vi "SRV_Determine Incoming Data Type.vi"(0 "Data":string, 11 "error in (no error)":errorcluster) -> (4 "Data dup":string, 10 "Response Data Type":T1=enum."No Data", 15 "error out":errorcluster)   [LabVIEW 2009]
doc: "Searches for identifying characters at the beginning of Data to determine the type of response the data is from.\n\n\nAuthor: Mike Schultz - Logic PD"
uses:
  SRV_Response Data Type.ctl
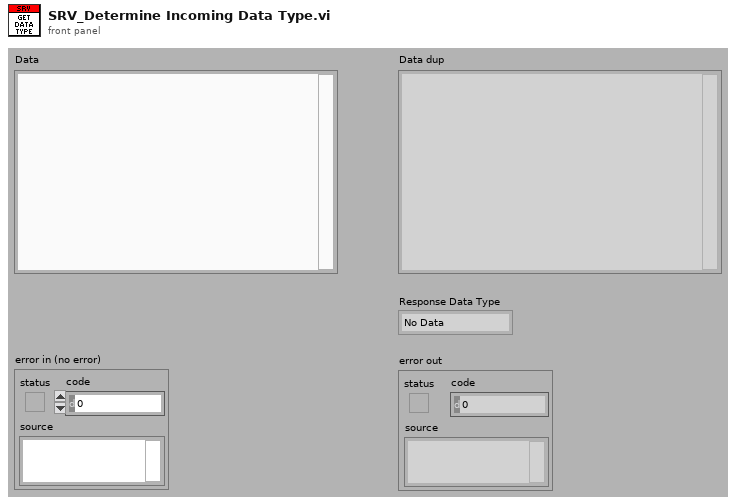
[diagram p1: front panel]
types:
  T1 = typedef "SRV_Response Data Type.ctl" = enum16{"Undefined Data", "##IMJ", "#B", "Leaving PicoC", "##vp", "##zZ", "##N$B", "##N$b", "##i$l", "##i$L", "##i$N", "##&NP,", "##&R,", "No Data"}
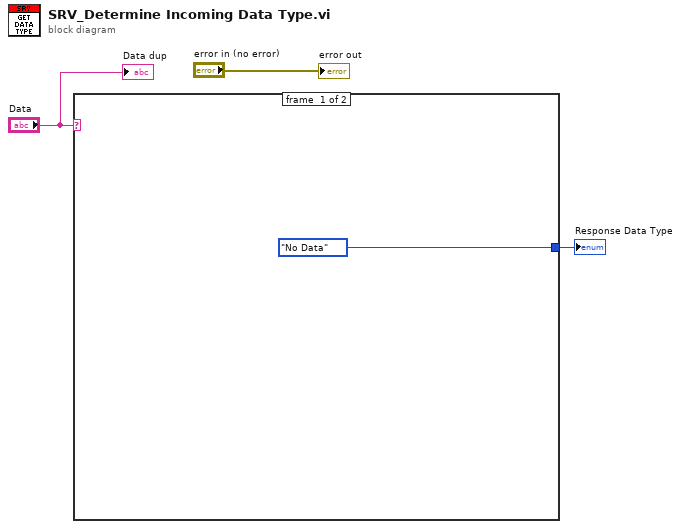
[diagram p0: block diagram]
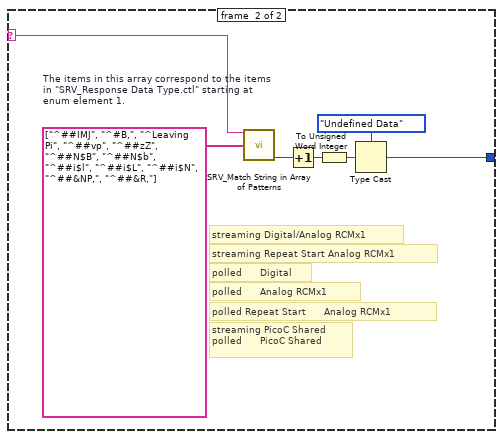
[diagram p2: hidden frame]
diagram:
  n1 = case shown="Default" "Data" {
    selector: "Data" -> [_ w10]
    tunnel: [SRV_Response_Data_Type."No Data" ("Response Data Type") w6] -> w3
    frame #0 {
    }
    frame #1 {
      w11 = string[] ["^##IMJ", "^#B,", "^Leaving Pi", "^##vp", "^##zZ", "^##N$B", "^##N$b", "^##i$l", "^##i$L", "^##i$N", "^##&NP,", "^##&R,"]  # The items in this array correspond to the items in "SRV_Response Data Type.ctl" starting at enum element 1.
      # "streaming Repeat Start Analog RCMx1"
      # "polled      Digital"
      # "polled Repeat Start      Analog RCMx1"
      # "streaming PicoC Shared\npolled      PicoC Shared"
      # "polled      Analog RCMx1"
      # "streaming Digital/Analog RCMx1"
      n2 = call "SRV_Match String in Array of Patterns.vi"("string"=w10, "regular expressions"=w11) -> ("index of Match"=w9:i32)  [unwired: 8 in, 5 out]
      n3 = Increment(x=w9) -> (x+1=w8:i32)
      n4 = To Unsigned Word Integer(number=w8) -> (unsigned 16bit integer=w7:u16)
      n5 = Type Cast(type=SRV_Response_Data_Type."Undefined Data" ("Response Data Type"), x=w7) -> (*(type *) &x=w6:T1)
    }
  }
  "Response Data Type" <- w3
  "Data dup" <- "Data"
  "error out" <- "error in (no error)"
